vi "DBedit_destructor.vi"(8 "error in (no error)":errorcluster, 11 "DB-editor in":refnum<class "DB-editor.lvclass">) -> (0 "error out":errorcluster, 3 "DB-editor out":refnum<class "DB-editor.lvclass">)   [LabVIEW 2020, in "Sgraph_lib_V1.lvlib" / "DB-editor.lvclass"]
doc: "Andre Koelewijn, 18 aug 2021\n\nEnd the Database editor application"
uses:
  DB-editor.lvclass
  Gserver/controls/Typedef_QueryType.ctl
  DB-editor.lvclass/DB-editor.ctl
  Gserver/Gserver.lvclass
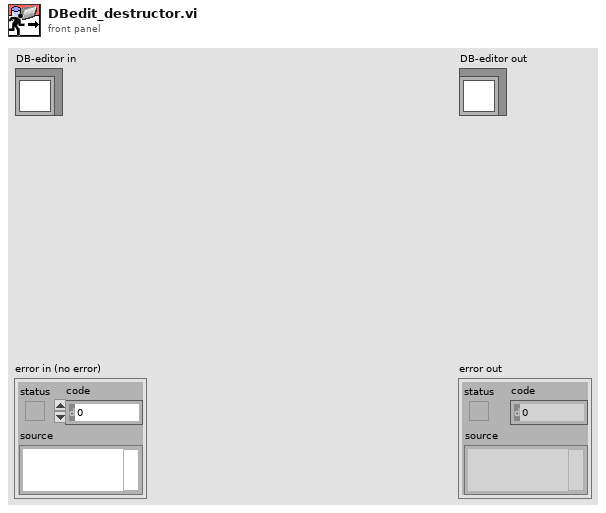
[diagram p1: front panel]
types:
  T1 = typedef "Sgraph_lib_V1.lvlib/Gserver.lvclass/Typedef_QueryType.ctl" = enum16{"Subscribe", "DataRequest", "RequestAllTags", "RequestIniPath", "FAMMstarted", "SetClientOptions", "GviewerUpdate", "OpenNewGraph", "CloseClient", "CloseAllClients", "Close Gserver", "OpenMemoryMap", "MeMapDataRequest", "MeMapDataResponse", "OpenDBeditor", "CheckDBeditorRunning", "StoppedDBeditor", "SaveDB_TAGpropRecord", "ConfirmDB_TAGpropSave"}
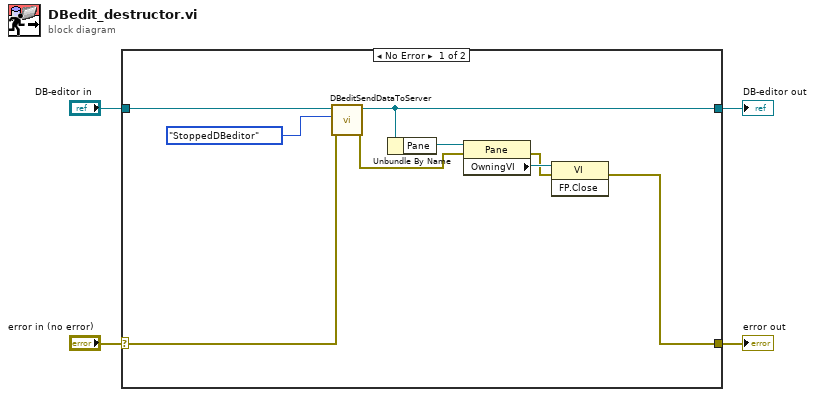
[diagram p0: block diagram]
diagram:
  n1 = case shown="No Error" "error in (no error)" {
    selector: "error in (no error)" -> [w11 w15]
    tunnel: [w5 w15] -> w3
    tunnel: [w10 w14] -> w1
    tunnel: "DB-editor in" -> [w12 w14]
    frame No Error {
      n2 = call "DBeditSendDataToServer.vi"("error in (no error)"=w11, "Query_type"=Typedef_QueryType."StoppedDBeditor", "Gviewer in"=w12) -> ("error out"=w6:errorcluster, "Gviewer out"=w10:refnum<class "DB-editor.lvclass">)  [unwired: 7 in]
      n3 = Unbundle By Name(w10) -> ("Pane"=w9:refnum<vi>)
      n4 = property class="Pane"(reference=w9, error in=w6) -> (error out=w7:errorcluster, "OwningVI"=w8:refnum<vi>)  [unwired: 1 out]
      n5 = invoke class="VI" method="FP.Close"(reference=w8, error in=w7) -> (error out=w5:errorcluster)  [unwired: 1 in, 2 out]
    }
    frame Error {
    }
  }
  "error out" <- w3
  "DB-editor out" <- w1
